vi "PreliminarySnakeCheck.vi"(8 "error in (no error)":errorcluster, 11 "Board in":T2[][](array[typedef])) -> (0 "error out":errorcluster, 1 "results":T1, 2 "tail position":cluster{"row":i32, "col":i32}, 3 "bodyparts set":set{cluster{i32, i32}}(c389))   [LabVIEW 2020]
uses:
  TypeDef/tiles-key-trunct.ctl
  88f61b10-d466-44c1-a86f-7e168586c36c.vi
  4b56118d-ba2a-410c-b4d4-3439df6b2749.vi
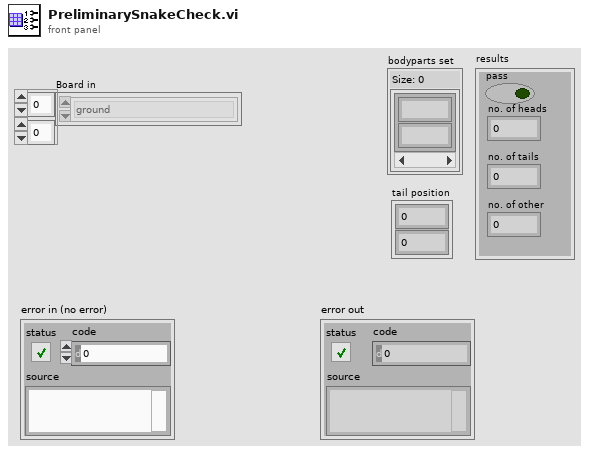
[diagram p1: front panel]
types:
  T1 = cluster{"pass":bool, "no. of heads":i32, "no. of tails":i32, "no. of other":i32}
  T2 = typedef "tiles-key-trunct.ctl" = enum16{"ground", "wall", "head (right)", "head (up)", "head (left)", "head (down)", "L-turn (right-up)", "L-turn (up-left)", "L-turn (left-down)", "L-turn (down-right)", "body (right)", "body (up)", "body (left)", "body (down)", "R-turn (right-down)", "R-turn (up-right)", "R-turn (left-up)", "R-turn (down-left)", "tail (right)", "tail (up)", "tail (left)", "tail (down)"}
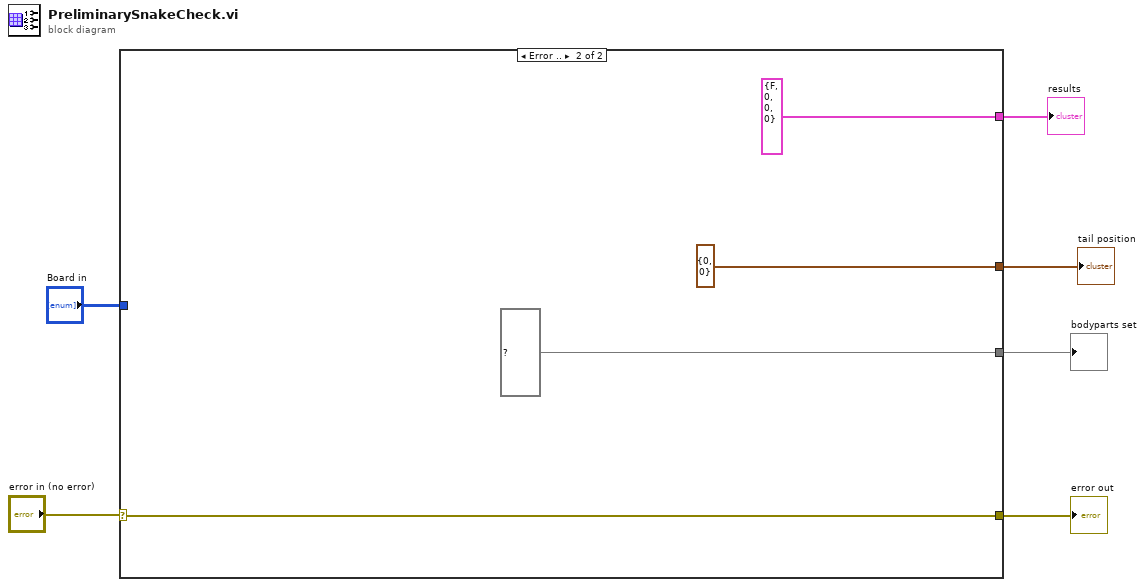
[diagram p0: block diagram]
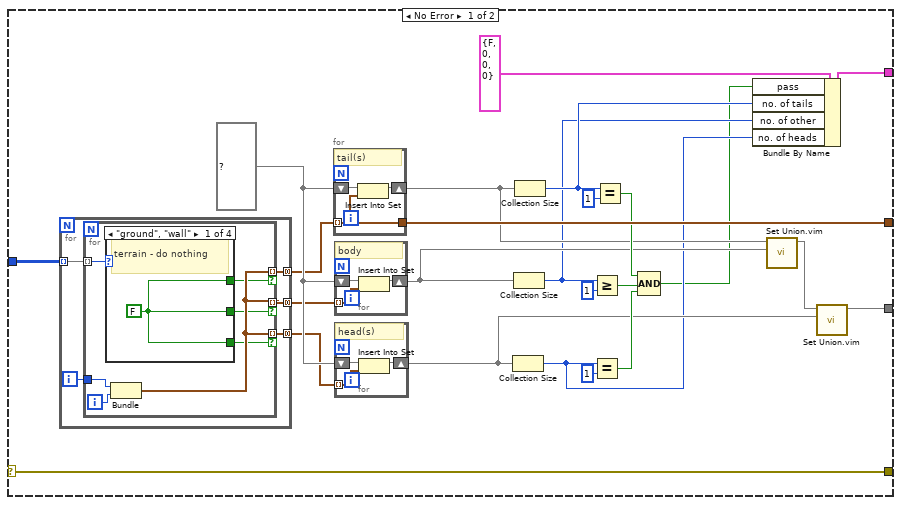
[diagram p2: hidden frame]
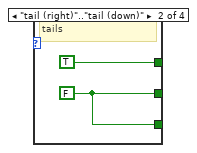
[diagram p3: hidden frame]
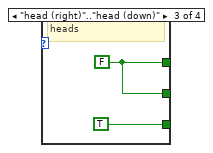
[diagram p4: hidden frame]
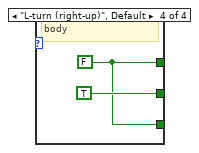
[diagram p5: hidden frame]
diagram:
  n1 = case shown="Error .." "error in (no error)" {
    selector: "error in (no error)" -> [w9 w59]
    tunnel: [w30 cluster{i32, i32} {0, 0}] -> w6
    tunnel: "Board in" -> [w29 _]
    tunnel: [w14 set{cluster{i32, i32}} {} ("union")] -> w4
    tunnel: [w13 T1 {"pass"=FALSE, "no. of heads"=0, "no. of tails"=0, "no. of other"=0} ("results")] -> w3
    tunnel: [w9 w59] -> w1
    frame No Error {
      w22 = set{cluster{i32, i32}} {} ("set in")
      n2 = for {
        tunnel: w29 -> [w44] mode=indexing
        tunnel: [w42] -> w19 mode=concatenating
        tunnel: [w41] -> w20 mode=concatenating
        tunnel: [w40] -> w21 mode=concatenating
        i -> [w43]
        n3 = for {
          tunnel: w44 -> [w51] mode=indexing
          tunnel: w43 -> [w49]
          tunnel: [w48] -> w42 mode=indexing if=w47
          tunnel: [w48] -> w41 mode=indexing if=w46
          tunnel: [w48] -> w40 mode=indexing if=w45
          i -> [w50]
          n4 = case shown="\"ground\", \"wall\"" w51 {
            tunnel: [w52 TRUE w55 w57] -> w47
            tunnel: [w52 w53 w55 TRUE] -> w46
            tunnel: [w52 w53 TRUE w57] -> w45
            frame "ground", "wall" {
              w52 = FALSE
              # "terrain - do nothing"
            }
            frame "tail (right)".."tail (down)" {
              w53 = FALSE
              # "tails"
            }
            frame "head (right)".."head (down)" {
              w55 = FALSE
              # "heads"
            }
            frame "L-turn (right-up)", Default {
              w57 = FALSE
              # "body"
            }
          }
          n5 = Bundle(w49, w50) -> (w48:cluster{i32, i32})  [unwired: 1 in]
        }
      }
      n6 = for {
        tunnel: w19 -> [w37] mode=indexing
        shift-right: [w38] -> w18
        shift-left: w22 -> [w39]
        tunnel: [w37] -> w30
        # "tail(s)"
        n7 = Insert Into Set(10:w37, 11:w39) -> (3:w38:set{cluster{i32, i32}})  [unwired: 1 out]
      }
      n8 = for {
        tunnel: w20 -> [w36] mode=indexing
        shift-right: [w34] -> w17
        shift-left: w22 -> [w35]
        # "body"
        n9 = Insert Into Set(10:w36, 11:w35) -> (3:w34:set{cluster{i32, i32}})  [unwired: 1 out]
      }
      n10 = for {
        tunnel: w21 -> [w33] mode=indexing
        shift-right: [w31] -> w15
        shift-left: w22 -> [w32]
        # "head(s)"
        n11 = Insert Into Set(10:w33, 11:w32) -> (3:w31:set{cluster{i32, i32}})  [unwired: 1 out]
      }
      n12 = Collection Size(1:w15) -> (0:w10:i32)
      n13 = Collection Size(1:w17) -> (0:w11:i32)
      n14 = Collection Size(1:w18) -> (0:w12:i32)
      n15 = Greater Or Equal?(x=w11, y=1) -> (x >= y?=w27:bool)
      n16 = Equal?(x=w10, y=1) -> (x = y?=w28:bool)
      n17 = Equal?(x=w12, y=1) -> (x = y?=w26:bool)
      n18 = Compound Arithmetic op=AND(w26, w27, w28) -> (w7:bool)
      n19 = Bundle By Name(cluster=T1 {"pass"=FALSE, "no. of heads"=0, "no. of tails"=0, "no. of other"=0} ("results"), "pass"=w7, "no. of tails"=w12, "no. of other"=w11, "no. of heads"=w10) -> (w13:T1)
      n20 = call "Set Union.vim"("set 2"=w17, "set 1"=w18) -> ("union"=w16:set{cluster{i32, i32}})  [unwired: 9 in]
      n21 = call "Set Union.vim"("set 2"=w15, "set 1"=w16) -> ("union"=w14:set{cluster{i32, i32}})  [unwired: 9 in]
    }
    frame Error {
    }
  }
  "tail position" <- w6
  "bodyparts set" <- w4
  "results" <- w3
  "error out" <- w1
